vi "ma_evalFormula.vi"(5 "t0":dbl format="%0.2f", 6 "Sampling info":cluster{"Fs":dbl, "#s":dbl}={"Fs"=1000.0, "#s"=1000.0} {"#s" format="%0.2p"; "Fs" format="%0.2p"}, 7 "Reset":bool, 8 "error in (no error)":errorcluster, 9 "Frequency":dbl format="%0.2f", 10 "Amplitude":dbl format="%0.2f", 11 "Formula":string) -> (0 "error out":errorcluster, 3 "Arbitrary Wave":dbl[](array[numeric]) format="%0.2f")   [LabVIEW 2020, in "NI_MAPro.lvlib"]
uses:
  NI_MAPro.lvlib
  NI_Gmath.lvlib
panel:
  in  "invalid variable name message":string="Invalid variable names.  Allowed variable names are: w, f, t, fs, a, or n"
  out "Waveform Graph":dbl[](graph)
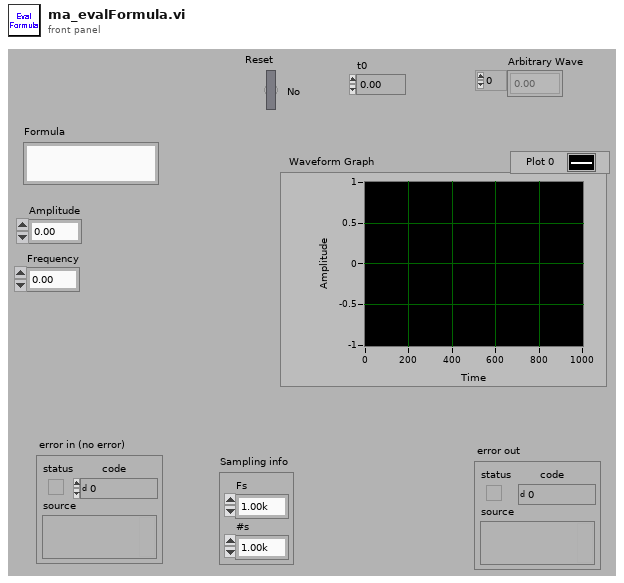
[diagram p1: front panel]
types:
  T1 = cluster{"parameter name":string, "parameter content":string}
  T2 = cluster{"parameter name":string, "parameter content":string}[]
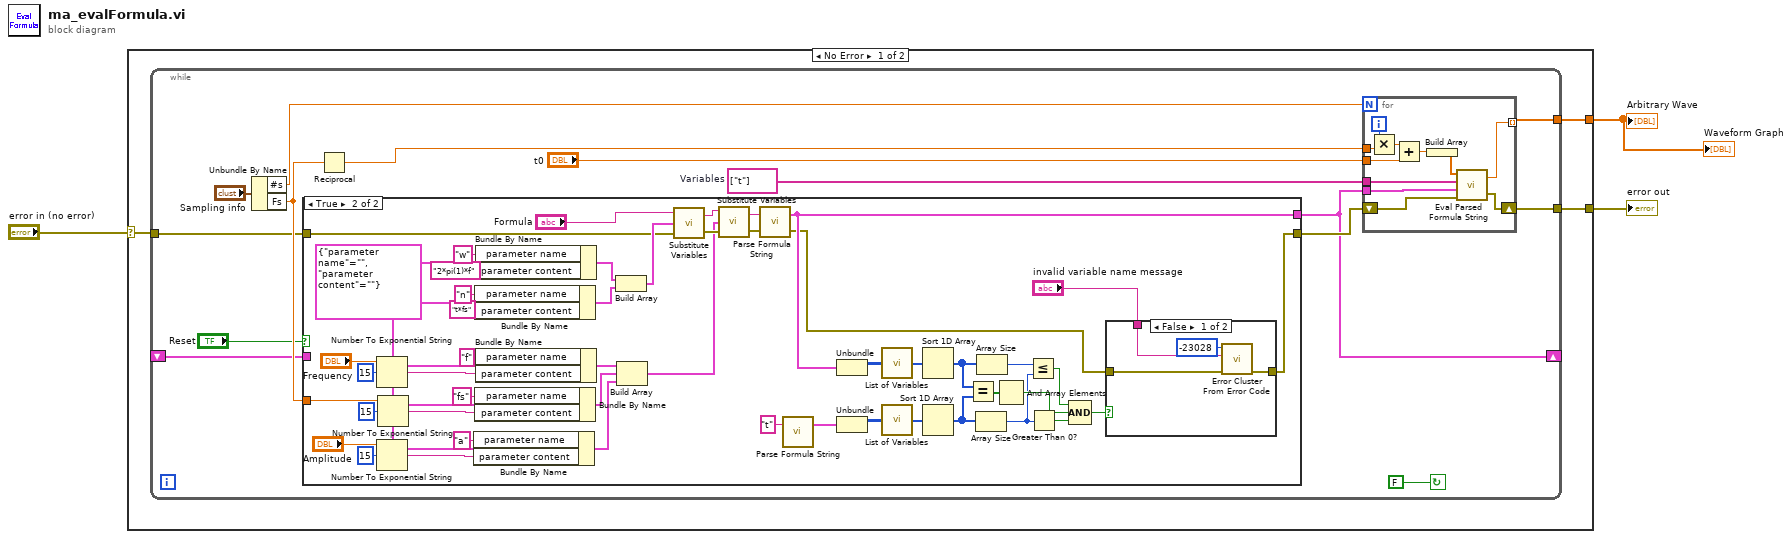
[diagram p0: block diagram]
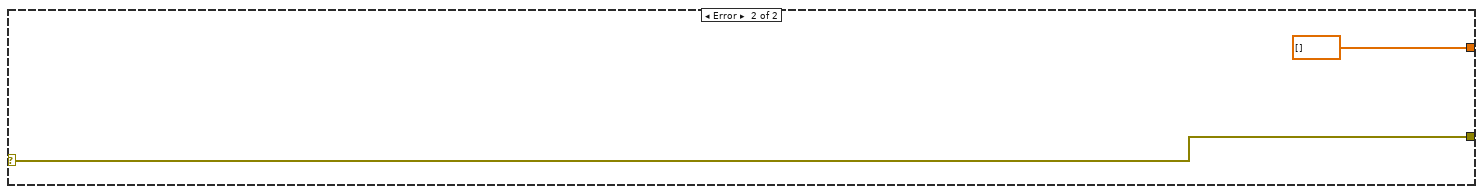
[diagram p4: hidden frame]
diagram:
  n1 = case shown="No Error" "error in (no error)" {
    selector: "error in (no error)" -> [w4 w88]
    tunnel: [w6 dbl[] []] -> w1
    tunnel: [w5 w88] -> w3
    frame No Error {
      n2 = while {
        tunnel: w4 -> [w11]
        shift-left: _ -> [w12]
        shift-right: [w13] -> _
        tunnel: [w8] -> w5
        tunnel: [w14] -> w6
        stop <- FALSE continue-if-true
        w9 = string[] ["t"]  # Variables
        n3 = Unbundle By Name("Sampling info") -> ("#s"=w16:dbl, "Fs"=w15:dbl)
        n4 = case shown="True" "Reset" {
          tunnel: [w21 w24] -> w19
          tunnel: [w22 w26] -> w13
          tunnel: w15 -> [_ w46]
          tunnel: w12 -> [w22 _]
          tunnel: w11 -> [w21 w42]
          frame False {
          }
          frame True {
            w43 = T1 {"parameter name"="", "parameter content"=""}
            n5 = Number To Exponential String(number="Frequency", 3:i16 15 ("width (-)")) -> (E-format string=w67:string)  [unwired: 2 out]
            n6 = Number To Exponential String(number="Amplitude", 3:i16 15 ("width (-)")) -> (E-format string=w56:string)  [unwired: 2 out]
            n7 = Number To Exponential String(number=w46, 3:i16 15 ("width (-)")) -> (E-format string=w61:string)  [unwired: 2 out]
            n8 = Bundle By Name(cluster=w43, "parameter name"="a" ("Bundle Element"), "parameter content"=w56) -> (w55:T1)
            n9 = Bundle By Name(cluster=w43, "parameter name"="n" ("Bundle Element"), "parameter content"="t*fs" ("Bundle Element")) -> (w49:T1)
            n10 = Bundle By Name(cluster=w43, "parameter name"="fs" ("Bundle Element"), "parameter content"=w61) -> (w63:T1)
            n11 = Bundle By Name(cluster=w43, "parameter name"="w" ("Bundle Element"), "parameter content"="2*pi(1)*f" ("Bundle Element")) -> (w68:T1)
            n12 = Bundle By Name(cluster=w43, "parameter name"="f" ("Bundle Element"), "parameter content"=w67) -> (w62:T1)
            n13 = Build Array(w68, w49) -> (w71:T2)
            n14 = Build Array(w62, w63, w55) -> (w48:T2)
            n15 = call "Substitute Variables.vi"("error in (no error)"=w42, "Substitution Rules"=w71, "original formula"="Formula") -> ("error out"=w69:errorcluster, "formula after substitution"=w70:string)
            n16 = call "Substitute Variables.vi"("error in (no error)"=w69, "Substitution Rules"=w48, "original formula"=w70) -> ("error out"=w53:errorcluster, "formula after substitution"=w52:string)
            n17 = call "Parse Formula String.vi"("error in (no error)"=w53, "formula"=w52) -> ("error out"=w25:errorcluster, "Parsed Formula"=w26:cluster{"Table":i32[][], "Y Values":dbl[]})
            n18 = call "Parse Formula String.vi"("formula"="t") -> ("Parsed Formula"=w37:cluster{"Table":i32[][], "Y Values":dbl[]})  [unwired: 1 in, 1 out]
            n19 = Unbundle(w26) -> ("Table"=w36:i32[][])  [unwired: 1 out]
            n20 = Unbundle(w37) -> ("Table"=w35:i32[][])  [unwired: 1 out]
            n21 = call "List of Variables.vi"("Table"=w36) -> ("List of variables"=w40:i32[])
            n22 = call "List of Variables.vi"("Table"=w35) -> ("List of variables"=w41:i32[])
            n23 = Sort 1D Array(array=w40) -> (sorted array=w30:i32[])
            n24 = Sort 1D Array(array=w41) -> (sorted array=w31:i32[])
            n25 = Equal?(x=w30, y=w31) -> (x = y?=w39:bool[])
            n26 = Array Size(array=w31) -> (size(s)=w28:i32)
            n27 = Array Size(array=w30) -> (size(s)=w29:i32)
            n28 = And Array Elements(Boolean array=w39) -> (logical AND=w38:bool)
            n29 = Less Or Equal?(x=w29, y=w28) -> (x <= y?=w33:bool)
            n30 = Greater Than 0?(x=w28) -> (x > 0?=w32:bool)
            n31 = Compound Arithmetic op=AND(w33, w38, w32) -> (w34:bool)
            n32 = case shown="False" w34 {
              tunnel: w25 -> [w74 w76]
              tunnel: [w73 w76] -> w24
              tunnel: "invalid variable name message" -> [w72 _]
              frame False {
                n33 = call "Error Cluster From Error Code.vi"("error in (no error)"=w74, "error message (\"\")"=w72, "error code (0)"=-23028) -> ("error out"=w73:errorcluster)  [unwired: 1 in, 5 out]
              }
              frame True {
              }
            }
          }
        }
        n34 = Reciprocal(x=w15) -> (1/x=w18:dbl)
        n35 = for {
          N: w16 -> [_]
          tunnel: w13 -> [w87]
          tunnel: w9 -> [w86]
          shift-right: [w84] -> w8
          shift-left: w19 -> [w85]
          tunnel: [w79] -> w14 mode=indexing
          tunnel: "t0" -> [w80]
          tunnel: w18 -> [w82]
          i -> [w83]
          n36 = Multiply(x=w83, y=w82) -> (x*y=w81:dbl)
          n37 = Add(x=w81, y=w80) -> (x+y=w77:dbl)
          n38 = Build Array(w77) -> (w78:dbl[])
          n39 = call "Eval Parsed Formula String.vi"("error in (no error)"=w85, "Parsed Formula"=w87, "Variables"=w86, "X Values"=w78) -> ("error out"=w84:errorcluster, "y value"=w79:dbl)
        }
      }
    }
    frame Error {
    }
  }
  "Arbitrary Wave" <- w1
  "error out" <- w3
  "Waveform Graph" <- w1
